vi "Setup.vi"(0 "SG Path Group in":refnum<class "SG Path Group.lvclass">, 11 "error in":errorcluster) -> (4 "SG Path Group out":refnum<class "SG Path Group.lvclass">, 15 "error out":errorcluster)   [LabVIEW 2023, in "RFFixtureCharact.RMM.lvlib" / "SG Path Group.lvclass"]
uses:
  SG Path Group.lvclass
  SG Path Group.lvclass/SG Path Group.ctl
  Instruments/Power Meter/Power Meter Factory/Power Meter Factory.lvclass
  Common/RFCalAndFixtureCharact.Common.lvlib
  Public/Base Classes/Scalar/SG Path/SG Path.lvclass
  Public/Base Classes/Scalar/Scalar Path/Scalar Path.lvclass
  Instruments/Power Meter/Power Meter Base/Power Meter Base.lvclass
  Public/Base Classes/Scalar/Scalar Path Group/Scalar Path Group.lvclass
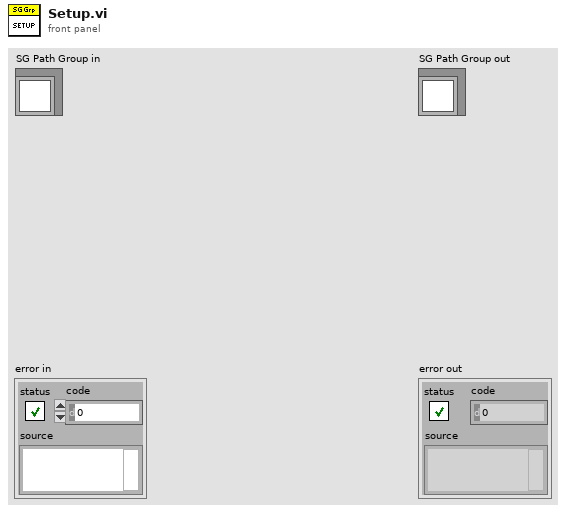
[diagram p1: front panel]
types:
  T1 = typedef "RFFixtureCharact.Public.lvlib/Scalar Path Group.lvclass/Sweep.ctl" = cluster{"Port Power":dbl, "Frequencies":dbl[], "Reference Level":dbl}
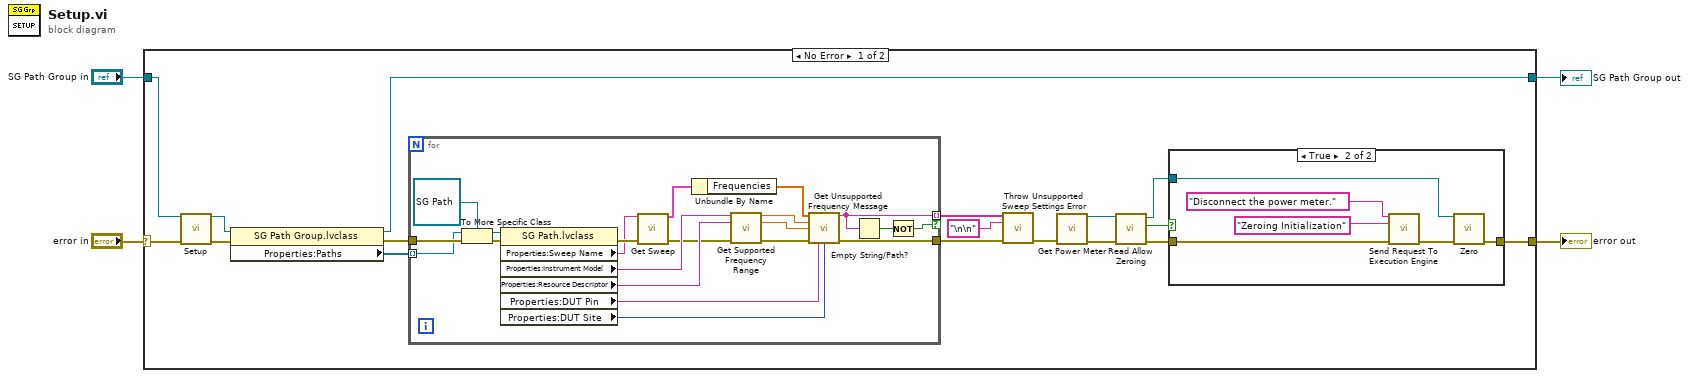
[diagram p0: block diagram]
diagram:
  n1 = case shown="No Error" "error in" {
    selector: "error in" -> [w21 w50]
    tunnel: [w19 w50] -> w3
    tunnel: "SG Path Group in" -> [w20 w51]
    tunnel: [w16 w51] -> w2
    frame No Error {
      n2 = call-parent "Setup.vi"("Path Group in"=w20, "error in"=w21) -> ("Path Group out"=w17:refnum<class "SG Path Group.lvclass">, "error out"=w18:errorcluster)  [unwired: 12 in]
      n3 = property class="SG Path Group.lvclass"(reference=w17, error in=w18) -> (reference out=w16:refnum<class "SG Path Group.lvclass">, error out=w14:errorcluster, "Properties:Paths"=w15:refnum<class "Path.lvclass">[])
      n4 = for {
        tunnel: w15 -> [w41] mode=indexing
        tunnel: w14 -> [w42]
        tunnel: [w35] -> w7
        tunnel: [w23] -> w5 mode=indexing if=w22
        n5 = To More Specific Class(target class=refnum<class "SG Path.lvclass"> refnum ("SG Path"), reference=w41, error in=w42) -> (specific class reference=w40:refnum<class "SG Path.lvclass">, error out=w39:errorcluster)
        n6 = property class="SG Path.lvclass"(reference=w40, error in=w39) -> (error out=w38:errorcluster, "Properties:Sweep Name"=w37:string, "Properties:Instrument Model"=w30:string, "Properties:Resource Descriptor"=w29:string, "Properties:DUT Pin"=w33:string, "Properties:DUT Site"=w32:i32)  [unwired: 1 out]
        n7 = call "Get Sweep.vi"("Sweep Name"=w37, "error in (no error)"=w38) -> ("Sweep"=w36:T1, "error out"=w28:errorcluster)  [unwired: 11 in, 1 out]
        n8 = Unbundle By Name(w36) -> ("Frequencies"=w34:dbl[])
        n9 = call "Get Supported Frequency Range.vi"("Instrument Model"=w30, "Instrument Name"=w29, "error in"=w28) -> ("Maximum Frequency"=w26:dbl, "Minmum Frequency"=w25:dbl, "error out"=w27:errorcluster)  [unwired: 10 in]
        n10 = call "Get Unsupported Frequency Message.vi"("Frequencies"=w34, "Maximum Frequency"=w26, "Minimum Frequency"=w25, "error in"=w27, "DUT Pin"=w33, "DUT Site"=w32) -> ("Unspported Frequency Message"=w23:string, "error out"=w35:errorcluster)  [unwired: 8 in]
        n11 = Empty String/Path?(string/path=w23) -> (empty?=w24:bool)
        n12 = Not(x=w24) -> (.not. x?=w22:bool)
      }
      n13 = call "Throw Unsupported Sweep Settings Error.vi"("Error Message List"=w5, "Paths Error Message Delimiter"="\n\n", "error in"=w7) -> ("error out"=w8:errorcluster)  [unwired: 12 in]
      n14 = call "Get Power Meter.vi"("error in (no error)"=w8) -> ("Power Meter Base out"=w13:refnum<class "Power Meter Base.lvclass">, "error out"=w12:errorcluster)  [unwired: 13 in]
      n15 = call-dynamic "Read Allow Zeroing.vi"("error in (no error)"=w12, "Power Meter Base in"=w13) -> ("error out"=w10:errorcluster, "Allow Zeroing"=w11:bool, "Power Meter Base out"=w9:refnum<class "Power Meter Base.lvclass">)  [unwired: 7 in]
      n16 = case shown="True" w11 {
        tunnel: w10 -> [w43 w47]
        tunnel: w9 -> [_ w46]
        tunnel: [w43 w44] -> w19
        frame False {
        }
        frame True {
          n17 = call "Send Request To Execution Engine.vi"("Request Message"="Disconnect the power meter." ("message"), "Request Header"="Zeroing Initialization", "error in (no error)"=w47) -> ("error out"=w45:errorcluster)  [unwired: 11 in, 1 out]
          n18 = call-dynamic "Zero.vi"("Power Meter Base in"=w46, "error in (no error)"=w45) -> ("error out"=w44:errorcluster)  [unwired: 12 in, 1 out]
        }
      }
    }
    frame Error {
    }
  }
  "error out" <- w3
  "SG Path Group out" <- w2
